vi "Next Lane.vi"(8 "error in (no error)":errorcluster, 11 "Stage Controller in":refnum<class "Stage Controller.lvclass">) -> (0 "error out":errorcluster, 3 "Stage Controller out":refnum<class "Stage Controller.lvclass">)   [LabVIEW 2018, in "Stage Controller.lvlib" / "Stage Controller.lvclass"]
uses:
  Stage Controller.lvclass
  Stage Controller.lvclass/Stage Controller.ctl
  <instrlib>/ASI TG-1000/Public/Utility/Axis Name.ctl
  Resources/GLOBAL/GLOBAL Debug.vi
  Microscope/ti2lv/ti2lv.lvlib
  <instrlib>/ASI TG-1000/ASI TG-1000.lvlib
  Stage Controller.lvlib
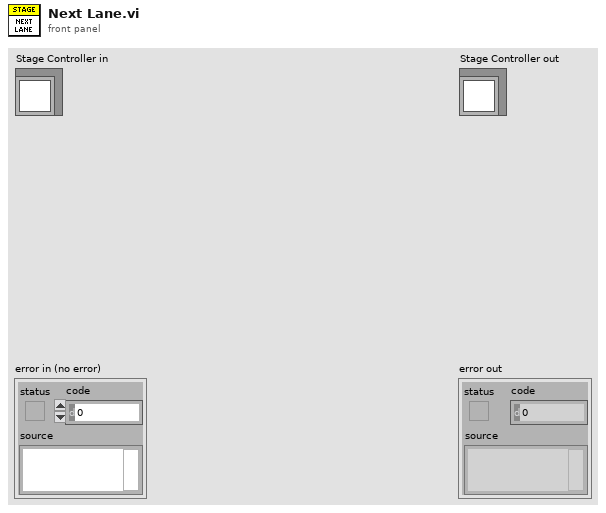
[diagram p1: front panel]
types:
  T1 = enum16{"Disabled", "ESP301", "Ti2", "Ludl", "ASI"}
  T2 = typedef "Stage Controller.lvlib/ASI TG-1000.lvlib/Axis Name.ctl" = enum8{"undefined", "A", "B", "C", "D", "E", "F", "G", "H", "I", "J", "K", "L", "M", "N", "O", "P", "Q", "R", "S", "T", "U", "V", "W", "X", "Y", "Z"}
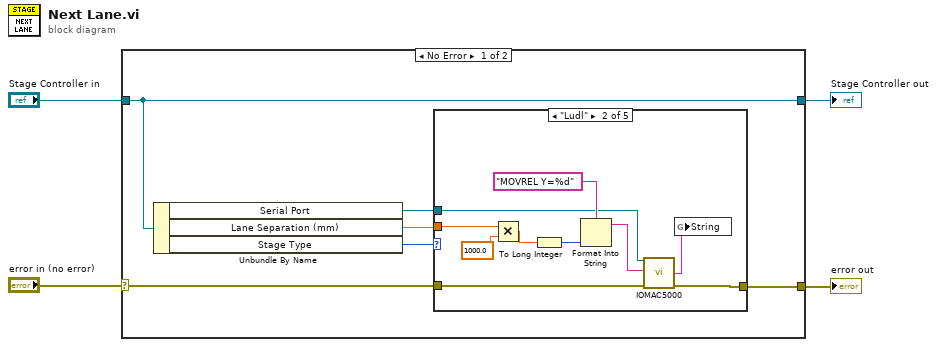
[diagram p0: block diagram]
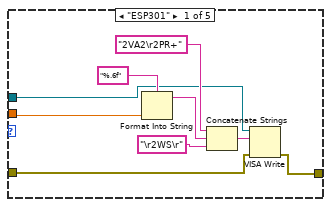
[diagram p2: hidden frame]
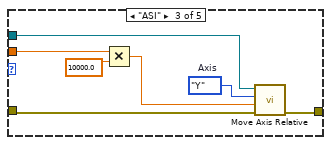
[diagram p3: hidden frame]
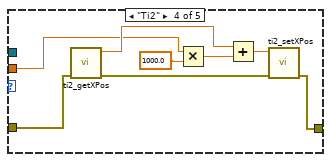
[diagram p4: hidden frame]
diagram:
  n1 = case shown="No Error" "error in (no error)" {
    selector: "error in (no error)" -> [w9 w47]
    tunnel: [w8 w47] -> w3
    tunnel: [w10 w46] -> w1
    tunnel: "Stage Controller in" -> [w10 w46]
    frame No Error {
      n2 = Unbundle By Name(w10) -> ("Serial Port"=w6:refnum<visa-resource-name>, "Lane Separation (mm)"=w7:dbl, "Stage Type"=w5:T1)
      n3 = case shown="\"Ludl\"" w5 {
        tunnel: w9 -> [w13 w23 w32 w44 w45]
        tunnel: [w14 w24 w33 w37 w45] -> w8
        tunnel: w7 -> [w11 w25 w31 w38 _]
        tunnel: w6 -> [w12 w21 w30 _ _]
        frame "ESP301" {
          n4 = Format Into String(format string="%.6f", w11) -> (resulting string=w18:string)  [unwired: 2 in, 1 out]
          n5 = Concatenate Strings("2VA2\r2PR+" ("write buffer"), w18, "\r2WS\r" ("write buffer")) -> (w19:string)
          n6 = VISA Write(VISA resource name=w12, write buffer=w19, error in (no error)=w13) -> (error out=w14:errorcluster)  [unwired: 2 out]
        }
        frame "Ludl" {
          n7 = Multiply(x=w25, y=1000.0) -> (x*y=w26:dbl)
          n8 = To Long Integer(number=w26) -> (32bit integer=w27:i32)
          n9 = Format Into String(format string="MOVREL Y=%d", w27) -> (resulting string=w22:string)  [unwired: 2 in, 1 out]
          n10 = call "IOMAC5000.vi"("VISA  IN"=w21, "Command (to ctlr)"=w22, "error in"=w23) -> ("Raw Response"=w20:string, "error out"=w24:errorcluster)  [unwired: 9 in, 2 out]
          n11 = global write "GLOBAL Debug.vi" "String"(w20) -> ()
        }
        frame "ASI" {
          w36 = Axis_Name."Y"  # Axis
          n12 = Multiply(x=w31, y=10000.0) -> (x*y=w35:dbl)
          n13 = call <instrlib>:"Move Axis Relative.vi"("error in (no error)"=w32, "Relative Position [internal units]"=w35, "Axis"=w36, "VISA in"=w30) -> ("error out"=w33:errorcluster)  [unwired: 5 in, 1 out]
        }
        frame "Ti2" {
          n14 = call "ti2_getXPos.vi"("error in (no error)"=w44) -> ("error out"=w43:errorcluster, "x Position (um)"=w39:dbl)  [unwired: 9 in]
          n15 = Multiply(x=w38, y=1000.0) -> (x*y=w40:dbl)
          n16 = Add(x=w39, y=w40) -> (x+y=w41:dbl)
          n17 = call "ti2_setXPos.vi"("error in (no error)"=w43, "x Position (um)"=w41) -> ("error out"=w37:errorcluster)  [unwired: 9 in]
        }
        frame "Disabled", Default {
        }
      }
    }
    frame Error {
    }
  }
  "error out" <- w3
  "Stage Controller out" <- w1
